vi "Breadth-first search day 16 fast index.vi"(9 "distance graph":T2(array[cluster]), 10 "Flow, bitfield":cluster{"flow":i32, "bitfield":u32}[](array[cluster]), 11 "input \n[index, bitfield, time left]":T1) -> (2 "most pressure":i32)   [LabVIEW 2023]
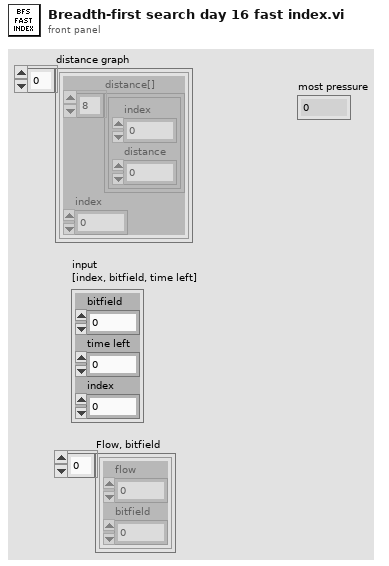
[diagram p1: front panel]
types:
  T1 = cluster{"bitfield":u32, "time left":i32, "index":i32}
  T2 = cluster{"distance[]":cluster{"index":i32, "distance":i32}[], "index":i32}[]
  T3 = cluster{"distance[]":cluster{"index":i32, "distance":i32}[], "index":i32}
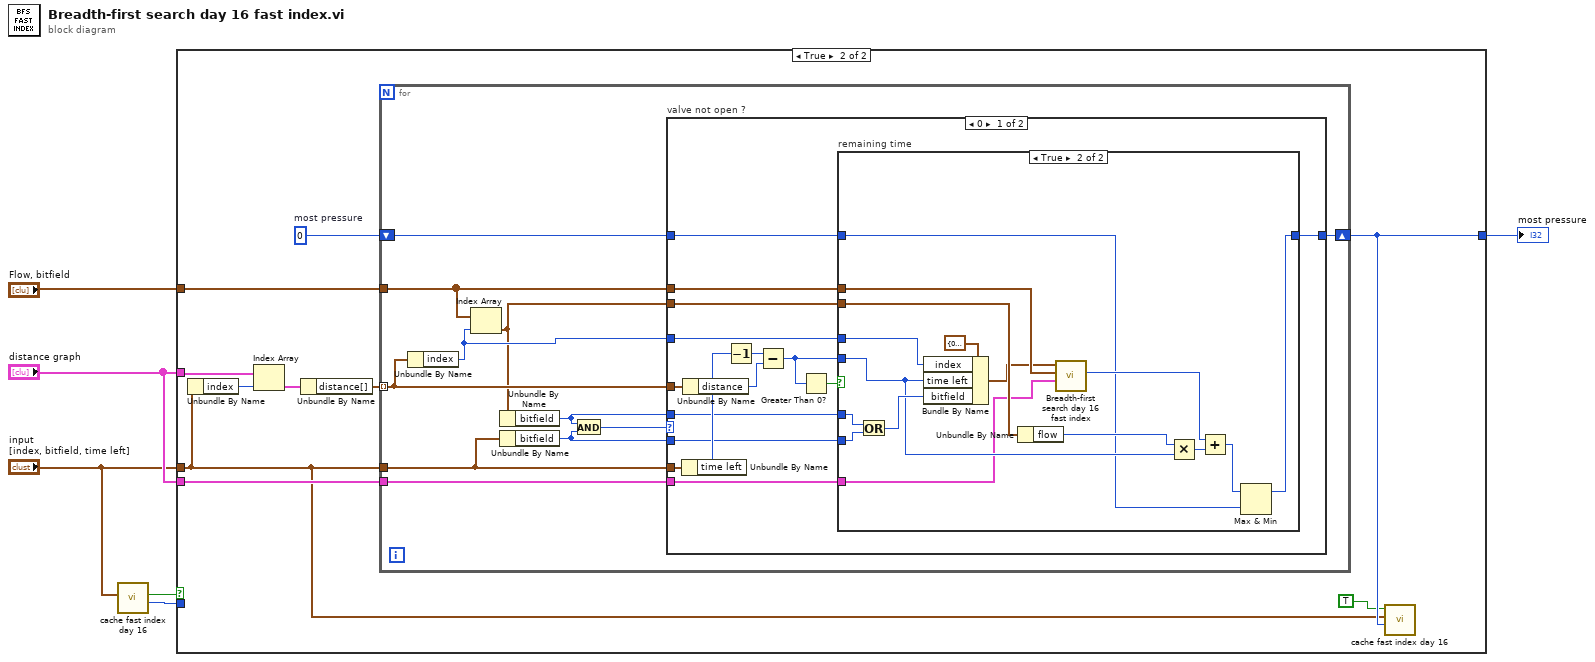
[diagram p0: block diagram]
diagram:
  n1 = call "cache fast index day 16.vi"("input \n[index, \nbitfield, \ntime left]"="input \n[index, bitfield, time left]") -> ("value"=w4:i32, "key not found?"=w5:bool)  [unwired: 9 in]
  n2 = case shown="True" w5 {
    tunnel: [w7 w16] -> w6
    tunnel: w4 -> [w7 _]
    tunnel: "distance graph" -> [_ w15]
    tunnel: "input \n[index, bitfield, time left]" -> [_ w9]
    tunnel: "Flow, bitfield" -> [_ w11]
    tunnel: "distance graph" -> [_ w10]
    frame False {
    }
    frame True {
      w17 = 0  # most pressure
      n3 = Unbundle By Name(w9) -> ("index"=w13:i32)
      n4 = Index Array(array=w15, index=w13) -> (element=w14:T3)
      n5 = Unbundle By Name(w14) -> ("distance[]"=w12:cluster{"index":i32, "distance":i32}[])
      n6 = for {
        shift-right: [w28] -> w16
        shift-left: w17 -> [w27]
        tunnel: w9 -> [w24]
        tunnel: w12 -> [w25] mode=indexing
        tunnel: w11 -> [w19]
        tunnel: w10 -> [w18]
        n7 = Unbundle By Name(w25) -> ("index"=w21:i32)
        n8 = Index Array(array=w19, index=w21) -> (element=w20:cluster{"flow":i32, "bitfield":u32})
        n9 = Unbundle By Name(w20) -> ("bitfield"=w22:u32)
        n10 = Unbundle By Name(w24) -> ("bitfield"=w23:u32)
        n11 = And(x=w22, y=w23) -> (x .and. y?=w26:u32)
        n12 = case "valve not open ?" shown="0" w26 {
          tunnel: [w43 w61] -> w28
          tunnel: w27 -> [w42 w61]
          tunnel: w25 -> [w39 _]
          tunnel: w24 -> [w38 _]
          tunnel: w23 -> [w34 _]
          tunnel: w22 -> [w33 _]
          tunnel: w21 -> [w32 _]
          tunnel: w20 -> [w31 _]
          tunnel: w19 -> [w30 _]
          tunnel: w18 -> [w29 _]
          frame 0 {
            n13 = Unbundle By Name(w38) -> ("time left"=w37:i32)
            n14 = Unbundle By Name(w39) -> ("distance"=w41:i32)
            n15 = Decrement(x=w37) -> (x-1=w40:i32)
            n16 = Subtract(x=w40, y=w41) -> (x-y=w35:i32)
            n17 = Greater Than 0?(x=w35) -> (x > 0?=w36:bool)
            n18 = case "remaining time" shown="True" w36 {
              tunnel: [w44 w45] -> w43
              tunnel: w42 -> [w44 w48]
              tunnel: w35 -> [_ w49]
              tunnel: w34 -> [_ w59]
              tunnel: w33 -> [_ w58]
              tunnel: w32 -> [_ w56]
              tunnel: w31 -> [_ w52]
              tunnel: w30 -> [_ w51]
              tunnel: w29 -> [_ w46]
              frame False {
              }
              frame True {
                n19 = Or(x=w58, y=w59) -> (x .or. y?=w57:u32)
                n20 = Bundle By Name(cluster=T1 {"bitfield"=0, "time left"=0, "index"=0}, "index"=w56, "time left"=w49, "bitfield"=w57) -> (w47:T1)
                n21 = Unbundle By Name(w52) -> ("flow"=w55:i32)
                n22 = call "Breadth-first search day 16 fast index.vi"("distance graph"=w46, "Flow, bitfield"=w51, "input \n[index, bitfield, time left]"=w47) -> ("most pressure"=w50:i32)  [unwired: 8 in]
                n23 = Multiply(x=w55, y=w49) -> (x*y=w53:i32)
                n24 = Add(x=w50, y=w53) -> (x+y=w54:i32)
                n25 = Max & Min(x=w54, y=w48) -> (max(x,y)=w45:i32)  [unwired: 1 out]
              }
            }
          }
          frame 1, Default {
          }
        }
      }
      n26 = call "cache fast index day 16.vi"("value"=w16, "input \n[index, \nbitfield, \ntime left]"=w9, "Add"=TRUE ("add")) -> ()  [unwired: 7 in, 2 out]
    }
  }
  "most pressure" <- w6
